vi "get.vi"(6 "request specific headers":T1[](array[typedef]), 7 "timeout (ms)":i32=10000, 8 "error in (no error)":errorcluster, 10 "path":string, 11 "reqwest in":refnum<class "reqwest.lvclass">) -> (0 "error out":errorcluster, 2 "response":string, 3 "reqwest out":refnum<class "reqwest.lvclass">)   [LabVIEW 2020, in "reqwest.lvclass"]
uses:
  reqwest.lvclass
  header.ctl
  reqwest.lvclass/reqwest.ctl
  shared-library/reqwest-labview.lvlib
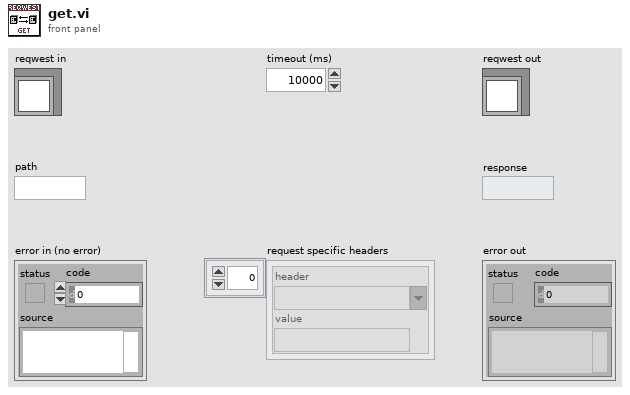
[diagram p1: front panel]
types:
  T1 = typedef "reqwest.lvclass/header.ctl" = cluster{"header":string, "value":string}
  T2 = typedef "reqwest.lvclass/private_data.ctl" = cluster{"Default Headers ([JSON])":T1[], "Base URL":string, "Authentication":cluster{"Username":string, "Password":string}}
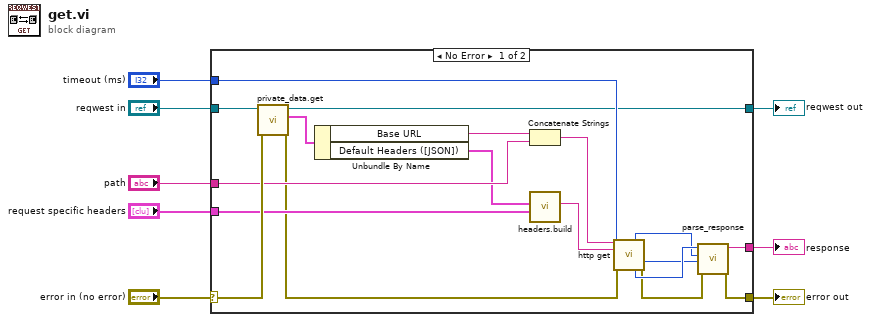
[diagram p0: block diagram]
diagram:
  n1 = case shown="No Error" "error in (no error)" {
    selector: "error in (no error)" -> [w25 w28]
    tunnel: [w10 w28] -> w7
    tunnel: [w15 w27] -> w5
    tunnel: "reqwest in" -> [w26 w27]
    tunnel: "path" -> [w22 _]
    tunnel: "request specific headers" -> [w20 _]
    tunnel: "timeout (ms)" -> [w16 _]
    tunnel: [w9 _] -> w2
    frame No Error {
      n2 = call "private_data.get.vi"("error in (no error)"=w25, "reqwest in"=w26) -> ("error out"=w17:errorcluster, "private data"=w24:T2, "reqwest out"=w15:refnum<class "reqwest.lvclass">)  [unwired: 7 in]
      n3 = Unbundle By Name(w24) -> ("Base URL"=w23:string, "Default Headers ([JSON])"=w21:T1[])
      n4 = Concatenate Strings(w23, w22) -> (w19:string)
      n5 = call "headers.build.vi"("request specific headers"=w20, "default headers"=w21) -> ("Headers JSON"=w18:string)  [unwired: 9 in]
      n6 = call "http get.vi"("url"=w19, "headers_json"=w18, "timeout_ms"=w16, "error in (no error)"=w17) -> ("response_len_out out"=w13:i32, "handle_out out"=w12:u64, "status_out out"=w14:u32, "error out"=w11:errorcluster)  [unwired: 7 in, 1 out]
      n7 = call "parse_response.vi"("error in"=w11, "handle_out"=w12, "response_len_out"=w13, "status_out"=w14) -> ("error out"=w10:errorcluster, "response"=w9:string)  [unwired: 6 in]
    }
    frame Error {
    }
  }
  "error out" <- w7
  "reqwest out" <- w5
  "response" <- w2
